vi "Change Version_VI Server Version.vi"() -> ()   [LabVIEW 2020, in "VI Server version.lvlib"]
uses:
  VI Server version.lvlib
  <vilib>/AppBuilder/AB_API_Simple/Build Specification Version.ctl
  <vilib>/AppBuilder/AB_API_Simple/NI_App_Builder_API.lvlib
panel:
  in  "Name of build specification":string="Exe"
  in  "Target Name (\"My Computer\" if empty)":string
  in  "Build Specification Version to set":T1
  out "error out":errorcluster
  out "Build Specification Version":T1
  # "Read first then write... so call twice to verify your change..."
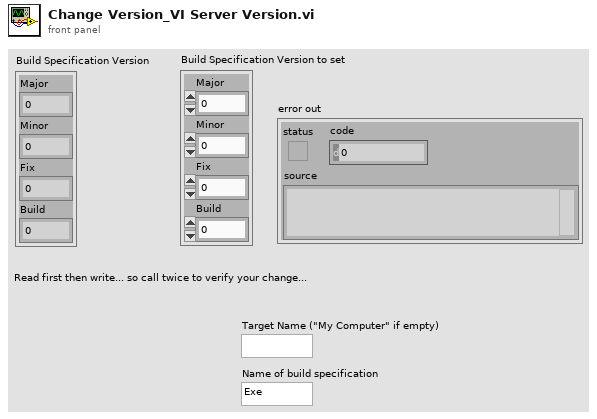
[diagram p1: front panel]
types:
  T1 = typedef "NI_App_Builder_API.lvlib/Build Specification Version.ctl" = cluster{"Major":u16, "Minor":u16, "Fix":u16, "Build":u16}
  T2 = cluster{"[0]":i32, "[1]":i32, "[2]":i32, "[3]":i32}
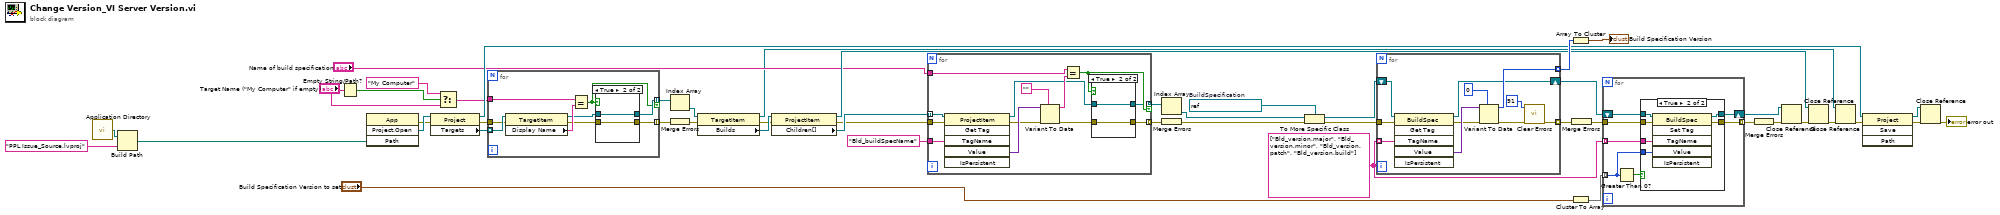
[diagram p0: block diagram]
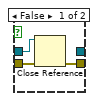
[diagram p2: hidden frame]
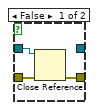
[diagram p3: hidden frame]
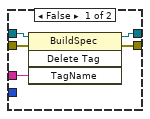
[diagram p4: hidden frame]
diagram:
  w36 = string[] ["Bld_version.major", "Bld_version.minor", "Bld_version.patch", "Bld_version.build"]
  w44 = refnum<vi> refnum  # BuildSpecification
  n1 = call <vilib>:"Application Directory.vi"() -> ("Application Directory"=w47:path)
  n2 = Build Path(base path=w47, name or relative path="PPL Issue_Source.lvproj") -> (appended path=w42:path)
  n3 = Empty String/Path?(string/path="Target Name (\"My Computer\" if empty)") -> (empty?=w10:bool)
  n4 = invoke class="App" method="Project.Open"("Path"=w42) -> (error out=w21:errorcluster, "Project:Open"=w41:refnum<vi>)  [unwired: 3 in, 2 out]
  n5 = property class="Project"(reference=w41, error in=w21) -> (reference out=w28:refnum<vi>, error out=w2:errorcluster, "Targets"=w5:refnum<vi>[])
  n6 = Select(t="My Computer", s=w10, f="Target Name (\"My Computer\" if empty)") -> (s? t:f=w7:string)
  n7 = for {
    tunnel: w5 -> [w57] mode=indexing
    tunnel: w7 -> [w55]
    tunnel: [w53] -> w6 mode=indexing if=w49
    tunnel: w2 -> [w52]
    tunnel: [w50] -> w3 mode=indexing
    n8 = property class="TargetItem"(reference=w57, error in=w52) -> (reference out=w54:refnum<vi>, error out=w51:errorcluster, "Display Name"=w56:string)
    n9 = Equal?(x=w55, y=w56) -> (x = y?=w49:bool)
    n10 = case shown="True" w49 {
      tunnel: [_ w62] -> w53
      tunnel: w54 -> [w60 w62]
      tunnel: w51 -> [w59 w61]
      tunnel: [w58 w61] -> w50
      frame False {
        n11 = Close Reference(reference=w60, error in (no error)=w59) -> (error out=w58:errorcluster)
      }
      frame True {
      }
    }
  }
  n12 = Index Array(array=w6) -> (element=w46:refnum<vi>)  [unwired: 1 in]
  n13 = Merge Errors(w3) -> (w1:errorcluster)
  n14 = property class="TargetItem"(reference=w46, error in=w1) -> (reference out=w4:refnum<vi>, error out=w22:errorcluster, "Builds"=w45:refnum<vi>)
  n15 = property class="ProjectItem"(reference=w45, error in=w22) -> (reference out=w32:refnum<vi>, error out=w13:errorcluster, "Children[]"=w18:refnum<vi>[])
  n16 = for {
    tunnel: w18 -> [w75] mode=indexing
    tunnel: "Bld_buildSpecName" ("String") -> [w74]
    tunnel: "Name of build specification" -> [w70]
    tunnel: w13 -> [w69]
    tunnel: [w66] -> w15 mode=indexing if=w68
    tunnel: [w63] -> w14 mode=indexing
    n17 = invoke class="ProjectItem" method="Get Tag"(reference=w75, error in=w69, "TagName"=w74) -> (reference out=w67:refnum<vi>, error out=w65:errorcluster, "Value"=w73:variant)  [unwired: 3 in, 3 out]
    n18 = Variant To Data(error in=w65, type="", Variant=w73) -> (data=w71:string, error out=w64:errorcluster)
    n19 = Equal?(x=w70, y=w71) -> (x = y?=w68:bool)
    n20 = case shown="True" w68 {
      tunnel: [_ w80] -> w66
      tunnel: w67 -> [w78 w80]
      tunnel: w64 -> [w77 w79]
      tunnel: [w76 w79] -> w63
      frame False {
        n21 = Close Reference(reference=w78, error in (no error)=w77) -> (error out=w76:errorcluster)
      }
      frame True {
      }
    }
  }
  n22 = Index Array(array=w15) -> (element=w43:refnum<vi>)  [unwired: 1 in]
  n23 = Merge Errors(w14) -> (w12:errorcluster)
  n24 = To More Specific Class(target class=w44, reference=w43, error in=w12) -> (specific class reference=w19:refnum<vi>, error out=w23:errorcluster)
  n25 = for {
    tunnel: w36 -> [w90] mode=indexing
    tunnel: [w87] -> w40 mode=indexing
    shift-right: [w86] -> w37
    shift-left: w19 -> [w91]
    tunnel: [w82] -> w25 mode=indexing
    tunnel: w23 -> [w83]
    n26 = invoke class="BuildSpec" method="Get Tag"(reference=w91, error in=w83, "TagName"=w90) -> (reference out=w86:refnum<vi>, error out=w85:errorcluster, "Value"=w89:variant)  [unwired: 3 in, 3 out]
    n27 = Variant To Data(error in=w85, type=0, Variant=w89) -> (data=w87:i32, error out=w84:errorcluster)
    n28 = call <vilib>:"Clear Errors.vi"("error in (no error)"=w84, "specific error code to clear (0: all)"=91) -> ("error out"=w82:errorcluster)  [unwired: 4 in, 1 out]
  }
  n29 = Array To Cluster(array=w40) -> (cluster=→"Build Specification Version":T2)
  n30 = Cluster To Array(cluster="Build Specification Version to set") -> (array=w35:u16[])
  n31 = Merge Errors(w25) -> (w24:errorcluster)
  n32 = for {
    tunnel: w36 -> [w97] mode=indexing
    shift-right: [w96] -> w11
    shift-left: w37 -> [w98]
    tunnel: w35 -> [w93] mode=indexing
    tunnel: [w95] -> w31 mode=indexing
    tunnel: w24 -> [w94]
    n33 = Greater Than 0?(x=w93) -> (x > 0?=w92:bool)
    n34 = case shown="True" w92 {
      tunnel: w98 -> [w103 w109]
      tunnel: w97 -> [w102 w108]
      tunnel: [w101 w107] -> w96
      tunnel: [w99 w106] -> w95
      tunnel: w94 -> [w100 w105]
      tunnel: w93 -> [_ w104]
      frame False {
        n35 = invoke class="BuildSpec" method="Delete Tag"(reference=w103, error in=w100, "TagName"=w102) -> (reference out=w101:refnum<vi>, error out=w99:errorcluster)  [unwired: 1 in, 2 out]
      }
      frame True {
        n36 = invoke class="BuildSpec" method="Set Tag"(reference=w109, error in=w105, "TagName"=w108, "Value"=w104) -> (reference out=w107:refnum<vi>, error out=w106:errorcluster)  [unwired: 2 in, 4 out]
      }
    }
  }
  n37 = Merge Errors(w31) -> (w30:errorcluster)
  n38 = Close Reference(reference=w11, error in (no error)=w30) -> (error out=w34:errorcluster)
  n39 = Close Reference(reference=w32, error in (no error)=w34) -> (error out=w33:errorcluster)
  n40 = Close Reference(reference=w4, error in (no error)=w33) -> (error out=w29:errorcluster)
  n41 = invoke class="Project" method="Save"(reference=w28, error in=w29) -> (reference out=w27:refnum<vi>, error out=w26:errorcluster)  [unwired: 2 in, 2 out]
  n42 = Close Reference(reference=w27, error in (no error)=w26) -> (error out=→"error out":errorcluster)
